vi "Return Front Panel State.vi"(8 "error in (no error)":errorcluster, 10 "State":T1(ring), 11 "reference":refnum<vi>) -> (0 "error out":errorcluster, 3 "reference out":refnum<vi>)   [LabVIEW 2015]
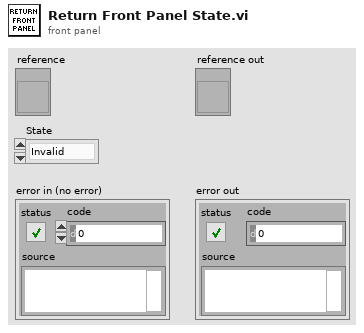
[diagram p1: front panel]
types:
  T1 = enum32{"Invalid", "Standard", "Closed", "Hidden", "Minimized", "Maximized"}
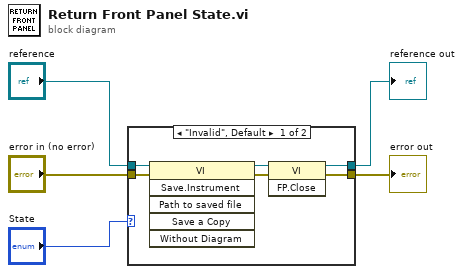
[diagram p0: block diagram]
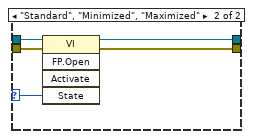
[diagram p2: hidden frame]
diagram:
  n1 = case shown="\"Invalid\", Default" "State" {
    selector: "State" -> [_ w12]
    tunnel: "error in (no error)" -> [w11 w16]
    tunnel: [w9 w15] -> w4
    tunnel: "reference" -> [w7 w14]
    tunnel: [w10 w13] -> w2
    frame "Invalid", Default {
      n2 = invoke class="VI" method="Save.Instrument"(reference=w7, error in=w11) -> (reference out=w6:refnum<vi>, error out=w8:errorcluster)  [unwired: 4 in, 4 out]
      n3 = invoke class="VI" method="FP.Close"(reference=w6, error in=w8) -> (reference out=w10:refnum<vi>, error out=w9:errorcluster)  [unwired: 1 in, 1 out]
    }
    frame "Standard", "Minimized", "Maximized" {
      n4 = invoke class="VI" method="FP.Open"(reference=w14, error in=w16, "State"=w12) -> (reference out=w13:refnum<vi>, error out=w15:errorcluster)  [unwired: 2 in, 3 out]
    }
  }
  "reference out" <- w2
  "error out" <- w4
